vi "GetSerializationDetails.vi"(8 "error in (no error)":errorcluster, 11 "VIConverter in":refnum<class "VIConverter.lvclass">) -> (0 "error out":errorcluster, 1 "ID":string, 2 "FileType":T1, 3 "VIConverter out":refnum<class "VIConverter.lvclass">, 4 "ComponentsSerialized":string)   [LabVIEW 2017, in "VIConverter.lvclass"]
uses:
  VIConverter.lvclass
  SupportedFileTypes.ctl
  GObjectConverters/FrontPanelConverter/FrontPanelConverter.lvclass
  GObjectConverters/DiagramConverter/DiagramConverter.lvclass
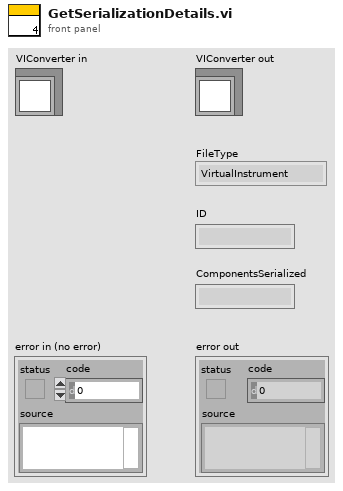
[diagram p1: front panel]
types:
  T1 = typedef "SupportedFileTypes.ctl" = enum16{"VirtualInstrument", "Polymorphic VI", "Class", "Project"}
  T2 = enum32{"invalid VI type", "Standard VI", "Control VI", "Global VI", "Polymorphic VI", "Configuration VI", "SubSystem", "Facade VI", "Method VI", "Statechart Diagram VI"}
  T3 = typedef "imagedata.ctl" = cluster{"image type":i32, "image depth":i32, "image":u8[], "mask":u8[], "colors":u32[], "Rectangle":cluster{"left":i16, "top":i16, "right":i16, "bottom":i16}}
  T4 = cluster{"VIPath":path, "Menu Name":string, "Selector Name":string}[]
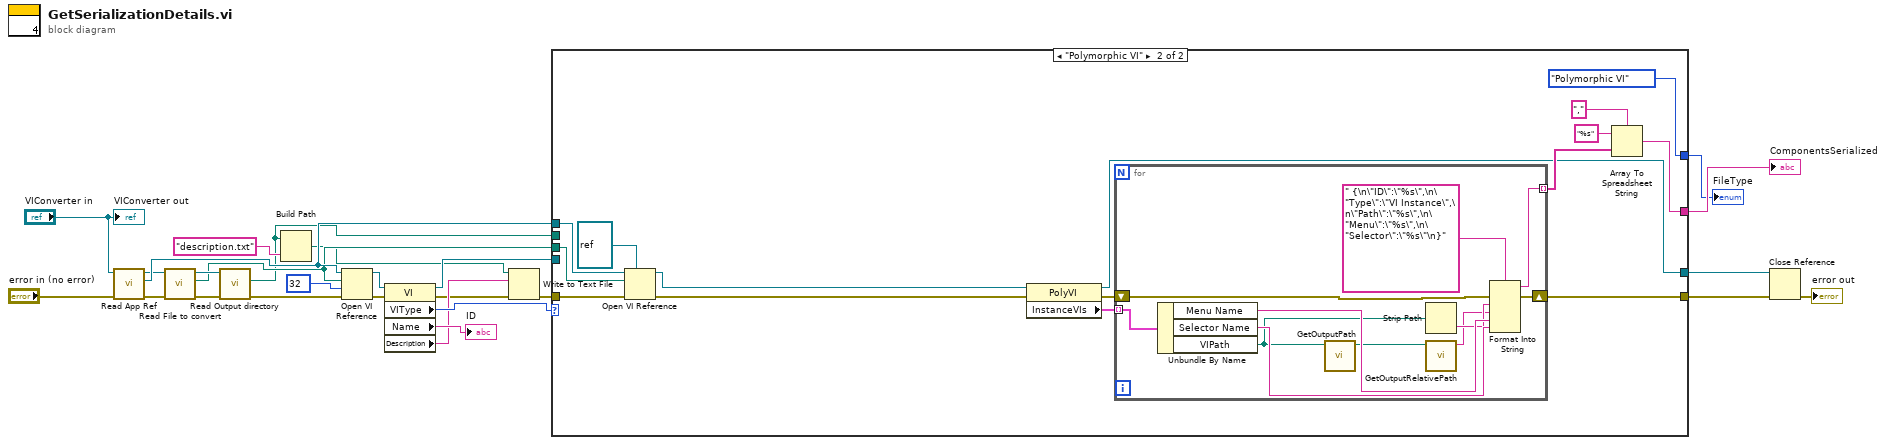
[diagram p0: block diagram]
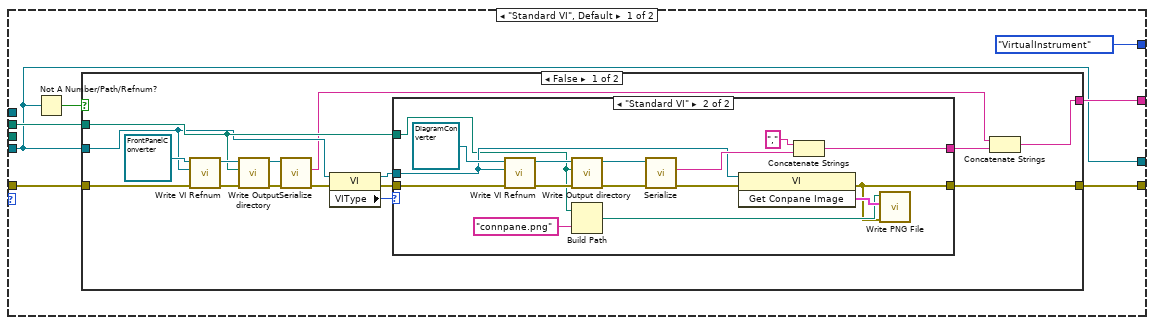
[diagram p2: hidden frame]
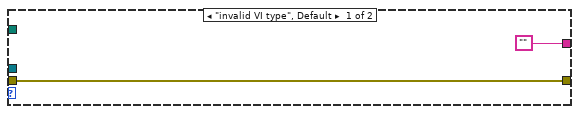
[diagram p3: hidden frame]
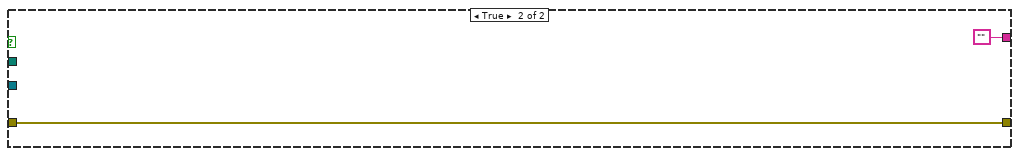
[diagram p4: hidden frame]
diagram:
  n1 = call-dynamic "Read App Ref.vi"("error in (no error)"="error in (no error)", "FileConverterBase in"="VIConverter in") -> ("error out"=w21:errorcluster, "App Ref"=w22:refnum<vi>, "FileConverterBase out"=w20:refnum<class "VIConverter.lvclass">)  [unwired: 7 in]
  n2 = call-dynamic "Read File to convert.vi"("error in (no error)"=w21, "FileConverterBase in"=w20) -> ("error out"=w19:errorcluster, "Input File Path"=w11:path, "FileConverterBase out"=w18:refnum<class "VIConverter.lvclass">)  [unwired: 7 in]
  n3 = call-dynamic "Read Output directory.vi"("error in (no error)"=w19, "FileConverterBase in"=w18) -> ("error out"=w17:errorcluster, "Output JSON File Path"=w1:path)  [unwired: 7 in, 1 out]
  n4 = Build Path(base path=w1, name or relative path="description.txt") -> (appended path=w7:path)
  n5 = Open VI Reference(application reference (local)=w22, vi path=w11, options=32, error in (no error)=w17) -> (vi reference=w25:refnum<vi>, error out=w12:errorcluster)  [unwired: 2 in]
  n6 = property class="VI"(reference=w25, error in=w12) -> (reference out=w9:refnum<vi>, error out=w5:errorcluster, "VIType"=w23:T2, "Name"=→"ID":string, "Description"=w6:string)
  n7 = Write to Text File(file (use dialog)=w7, text=w6, error in=w5) -> (error out=w4:errorcluster)  [unwired: 1 in, 2 out]
  n8 = case shown="\"Polymorphic VI\"" w23 {
    tunnel: w4 -> [w32 w77]
    tunnel: w9 -> [w27 _]
    tunnel: w22 -> [_ w76]
    tunnel: [w31 w75] -> w15
    tunnel: w1 -> [w29 _]
    tunnel: w11 -> [_ w73]
    tunnel: [SupportedFileTypes."VirtualInstrument" ("Supported File Types") SupportedFileTypes."Polymorphic VI" ("Supported File Types")] -> w10
    tunnel: [w28 w71] -> w3
    tunnel: [w27 w70] -> w2
    frame "Standard VI", Default {
      n9 = Not A Number/Path/Refnum?(number/path/refnum=w27) -> (NaN/Path/Refnum?=w33:bool)
      n10 = case shown="False" w33 {
        tunnel: [w44 w69] -> w28
        tunnel: w32 -> [w37 w69]
        tunnel: w27 -> [w42 _]
        tunnel: [w39 ""] -> w31
        tunnel: w29 -> [w43 _]
        frame False {
          n11 = call-dynamic "Write VI Refnum.vi"("error in (no error)"=w37, "VI Refnum"=w42, "VIObjectConverter in"=refnum<class "FrontPanelConverter.lvclass"> refnum ("FrontPanelConverter.lvclass")) -> ("error out"=w47:errorcluster, "VIObjectConverter out"=w46:refnum<class "FrontPanelConverter.lvclass">)  [unwired: 7 in]
          n12 = call-dynamic "Write Output directory.vi"("error in (no error)"=w47, "Output directory"=w43, "GObjectConverterBase in"=w46) -> ("error out"=w48:errorcluster, "GObjectConverterBase out"=w49:refnum<class "FrontPanelConverter.lvclass">)  [unwired: 7 in]
          n13 = call-dynamic "Serialize.vi"("error in (no error)"=w48, "FrontPanelConverter in"=w49) -> ("error out"=w36:errorcluster, "JSON"=w40:string)  [unwired: 7 in, 1 out]
          n14 = property class="VI"(reference=w42, error in=w36) -> (reference out=w41:refnum<vi>, error out=w35:errorcluster, "VIType"=w34:T2)
          n15 = case shown="\"Standard VI\"" w34 {
            tunnel: w41 -> [_ w57]
            tunnel: ["" w59] -> w38
            tunnel: [w50 w52] -> w44
            tunnel: w43 -> [_ w54]
            tunnel: w35 -> [w50 w62]
            frame "invalid VI type", Default {
            }
            frame "Standard VI" {
              n16 = call-dynamic "Write VI Refnum.vi"("error in (no error)"=w62, "VI Refnum"=w57, "VIObjectConverter in"=refnum<class "DiagramConverter.lvclass"> refnum ("DiagramConverter.lvclass")) -> ("error out"=w66:errorcluster, "VIObjectConverter out"=w67:refnum<class "DiagramConverter.lvclass">)  [unwired: 7 in]
              n17 = call-dynamic "Write Output directory.vi"("error in (no error)"=w66, "Output directory"=w54, "GObjectConverterBase in"=w67) -> ("error out"=w65:errorcluster, "GObjectConverterBase out"=w64:refnum<class "DiagramConverter.lvclass">)  [unwired: 7 in]
              n18 = Build Path(base path=w54, name or relative path="connpane.png") -> (appended path=w56:path)
              n19 = call-dynamic "Serialize.vi"("error in (no error)"=w65, "DiagramConverter in"=w64) -> ("error out"=w53:errorcluster, "JSON"=w61:string)  [unwired: 7 in, 1 out]
              n20 = invoke class="VI" method="Get Conpane Image"(reference=w57, error in=w53) -> (error out=w52:errorcluster, "Get Conpane Image"=w58:T3)  [unwired: 1 in, 1 out]
              n21 = Concatenate Strings("," ("string"), w61) -> (w59:string)
              n22 = call <vilib>:"Write PNG File.vi"("error in (no error)"=w52, "image data"=w58, "path to PNG file"=w56) -> ()  [unwired: 7 in, 2 out]
            }
          }
          n23 = Concatenate Strings(w40, w38) -> (w39:string)
        }
        frame True {
        }
      }
    }
    frame "Polymorphic VI" {
      n24 = Open VI Reference(type specifier VI Refnum (for type only)=refnum<vi> refnum, application reference (local)=w76, vi path=w73, error in (no error)=w77) -> (vi reference=w83:refnum<vi>, error out=w74:errorcluster)  [unwired: 2 in]
      n25 = property class="PolyVI"(reference=w83, error in=w74) -> (reference out=w70:refnum<vi>, error out=w78:errorcluster, "InstanceVIs"=w82:T4)
      n26 = for {
        tunnel: w82 -> [w95] mode=indexing
        tunnel: [w92] -> w81 mode=indexing
        shift-right: [w90] -> w71
        shift-left: w78 -> [w89]
        n27 = Unbundle By Name(w95) -> ("Menu Name"=w94:string, "Selector Name"=w93:string, "VIPath"=w85:path)
        n28 = call "GetOutputPath.vi"("Path"=w85) -> ("Output Path"=w87:path)  [unwired: 10 in]
        n29 = Strip Path(path=w85) -> (name=w91:string)  [unwired: 1 out]
        n30 = call "GetOutputRelativePath.vi"("Path"=w87) -> ("Output relative path"=w86:string)  [unwired: 9 in, 1 out]
        n31 = Format Into String(format string=" {\n\"ID\":\"%s\",\n\"Type\":\"VI Instance\",\n\"Path\":\"%s\",\n\"Menu\":\"%s\",\n\"Selector\":\"%s\"\n}", error in=w89, w91, w86, w94, w93) -> (resulting string=w92:string, error out=w90:errorcluster)  [unwired: 1 in]
      }
      n32 = Array To Spreadsheet String(delimiter (Tab)=",", array=w81, 3:"%s" ("format string")) -> (spreadsheet string=w75:string)
    }
  }
  "FileType" <- w10
  "ComponentsSerialized" <- w15
  n33 = Close Reference(reference=w2, error in (no error)=w3) -> (error out=→"error out":errorcluster)
  "VIConverter out" <- "VIConverter in"
